vi "StartTest.vi"(8 "error in (no error)":errorcluster, 10 "SeqExeQuueIn":refnum<queue>, 11 "TestSeqClass in":refnum<class "TestSeqClass.lvclass">) -> (0 "error out":errorcluster, 3 "TestSeqClass out":refnum<class "TestSeqClass.lvclass">)   [LabVIEW 2019, in "TestSeqClass.lvclass"]
uses:
  TestSeqClass.lvclass
  TestSeqClass.lvclass/TestSeqClass.ctl
  Write CurrentTestPointer.vi
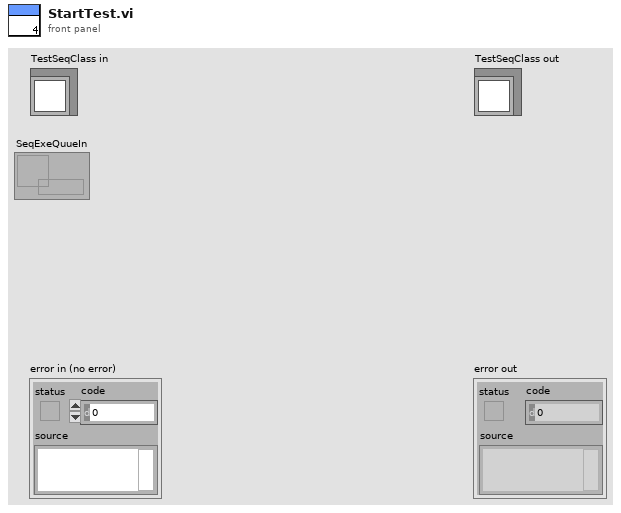
[diagram p1: front panel]
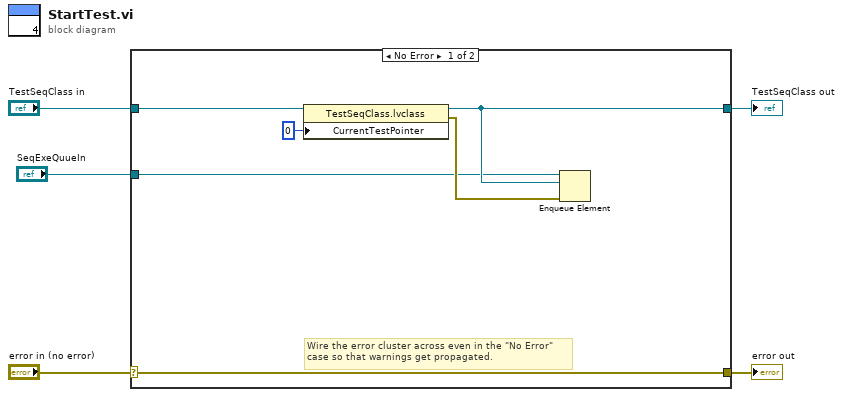
[diagram p0: block diagram]
diagram:
  n1 = case shown="No Error" "error in (no error)" {
    selector: "error in (no error)" -> [w11 w13]
    tunnel: [w11 w13] -> w4
    tunnel: [w8 w12] -> w2
    tunnel: "TestSeqClass in" -> [w10 w12]
    tunnel: "SeqExeQuueIn" -> [w6 _]
    frame No Error {
      # "Wire the error cluster across even in the \"No Error\"\ncase so that warnings get propagated."
      n2 = property class="TestSeqClass.lvclass"(reference=w10, "CurrentTestPointer"=u32 0) -> (reference out=w8:refnum<class "TestSeqClass.lvclass">, error out=w7:errorcluster)  [unwired: 1 in]
      n3 = Enqueue Element(queue=w6, element=w8, error in (no error)=w7) -> ()  [unwired: 1 in, 3 out]
    }
    frame Error {
    }
  }
  "error out" <- w4
  "TestSeqClass out" <- w2
